vi "Actor Core.vi"(8 "error in":errorcluster, 11 "gController in":refnum<class "gController.lvclass">) -> (0 "error out":errorcluster, 3 "Actor out":refnum<class "Actor.lvclass">)   [LabVIEW 2017, in "Controller.lvlib" / "gController.lvclass"]
doc: "(<B>Filename</B>: Actor Framework.lvlib:Actor.lvclass:Actor Core.vi)\n\nReceives messages to the actor, reacts to them, and initiates any error handling that may shut the actor down.\n\nDescendant classes may override this VI to append parallel tasks for the actor to complete while it handles messages. Overrides use the Call Parent Method node."
uses:
  gController.lvclass
  C:/Program Files (x86)/National Instruments/LabVIEW 2017/vi.lib/MSR Consulting, LLC/General Reuse/SuperActor/SuperActor.lvclass
  <vilib>/ActorFramework/Actor/Actor.lvclass
  File Actor/File Actor.lvclass
  C:/Program Files (x86)/National Instruments/LabVIEW 2017/vi.lib/ActorFramework/Actor/Actor.lvclass
  File Actor/Messages/Abstract/Saving File Message/Saving File Message.lvclass
  Commands/Exe Write Main CMD/Exe Write Main CMD.lvclass
  G:/sw_repo/For Builds/Nicholas/File Actor/Messages/Abstract/Exe Write/Exe Write.lvclass
  <vilib>/ActorFramework/Message Enqueuer/Message Enqueuer.lvclass
  <vilib>/Platform/TimedLoop/XDataNode/timing_clust.ctl
  <vilib>/Platform/TimedLoop/XDataNode/nitl_modes.ctl
  <vilib>/Platform/TimedLoop/XDataNode/wakeup.ctl
  <vilib>/MSR Consulting, LLC/General Reuse/SuperActor/SuperActor.lvclass/SuperActor.ctl
  gController.lvclass/gController.ctl
  Commands/Exe Write Main CMD/Exe Write Main CMD.lvclass/Exe Write Main CMD.ctl
  File Actor/File Actor.lvclass/File Actor.ctl
  File Actor/Messages/To/Data/File Data Message.lvclass
  C:/Program Files (x86)/National Instruments/LabVIEW 2017/vi.lib/ActorFramework/Message/Message.lvclass
  <vilib>/ActorFramework/Message Enqueuer/Message Enqueuer.lvclass/Message Enqueuer.ctl
  File Actor/Write Saving FIle MSG.vi
  File Actor/Write Exe Write.vi
  <vilib>/MSR Consulting, LLC/General Reuse/SuperActor/Write ID.vi
  File Actor/Write Cfg Header.vi
  File Actor/Write Wait on Registration_.vi
  <vilib>/MSR Consulting, LLC/General Reuse/SuperActor/Read Log Session.vi
  Read DataMap.vi
  Commands/Exe Write Main CMD/Write DataMap.vi
  <vilib>/MSR Consulting, LLC/General Reuse/SuperActor/Read EnqueuerMap.vi
  <vilib>/ActorFramework/Message Priority Queue/Priority Enqueue.vi
  File Actor/Write Registration Complete.vi
  <vilib>/Platform/TimedLoop/XDataNode/XDataNode.xnode
  <vilib>/MSR Consulting, LLC/General Reuse/Session APIs/_Session Fwk/Session - Root.lvclass
  <vilib>/MSR Consulting, LLC/General Reuse/SuperActor/SuperActor.lvclass
  <vilib>/MSR Consulting, LLC/General Reuse/Session APIs/Session Log/System Log.lvclass
  <vilib>/Platform/TimedLoop/XDataNode/XDNodeRunTimeDep.lvlib
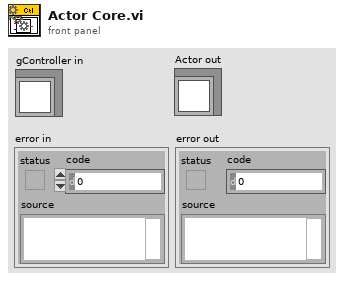
[diagram p1: front panel]
types:
  T1 = typedef "Session - Root.lvclass/Session Handle.ctl" = refnum<data-value>
  T2 = typedef "XDNodeRunTimeDep.lvlib/timing_clust.ctl" = cluster{"Expected End [f-1]":u64, "Actual End [f-1]":u64, "Finished Late? [f-1]":bool, "Expected End [i-1]":u64, "Actual End [i-1]":u64, "Finished Late? [i-1]":bool, "Expected Start [i]":u64, "Actual Start [i]":u64, "Expected Start [f]":u64, "Actual Start [f]":u64, "Source Name":string, "Structure Name":string, "Period":i64, "Deadline":i64, "Offset":i64, "Start":i64, "Priority":i32, "Timeout":i32, "Mode":T3, "Wakeup Reason":T4, "Error":errorcluster, "Source Type":string, "Secondary Source Type":string, "Global End Time":u64, "Global Start Time":u64, "Frame Duration":u64, "Iteration Duration":u64, "Assigned CPU":i32, "I/O Scan Engine Mode":u32}
  T3 = typedef "XDNodeRunTimeDep.lvlib/nitl_modes.ctl" = enum32{"No Change", "Process missed periods, maintain original phase", "Discard missed periods, maintain original phase", "Process missed periods, ignore original phase", "Discard missed periods, ignore original phase"}
  T4 = typedef "XDNodeRunTimeDep.lvlib/wakeup.ctl" = enum32{"Normal", "Aborted", "Asynchronous wakeup", "Timing source error", "Timed loop error", "Timeout"}
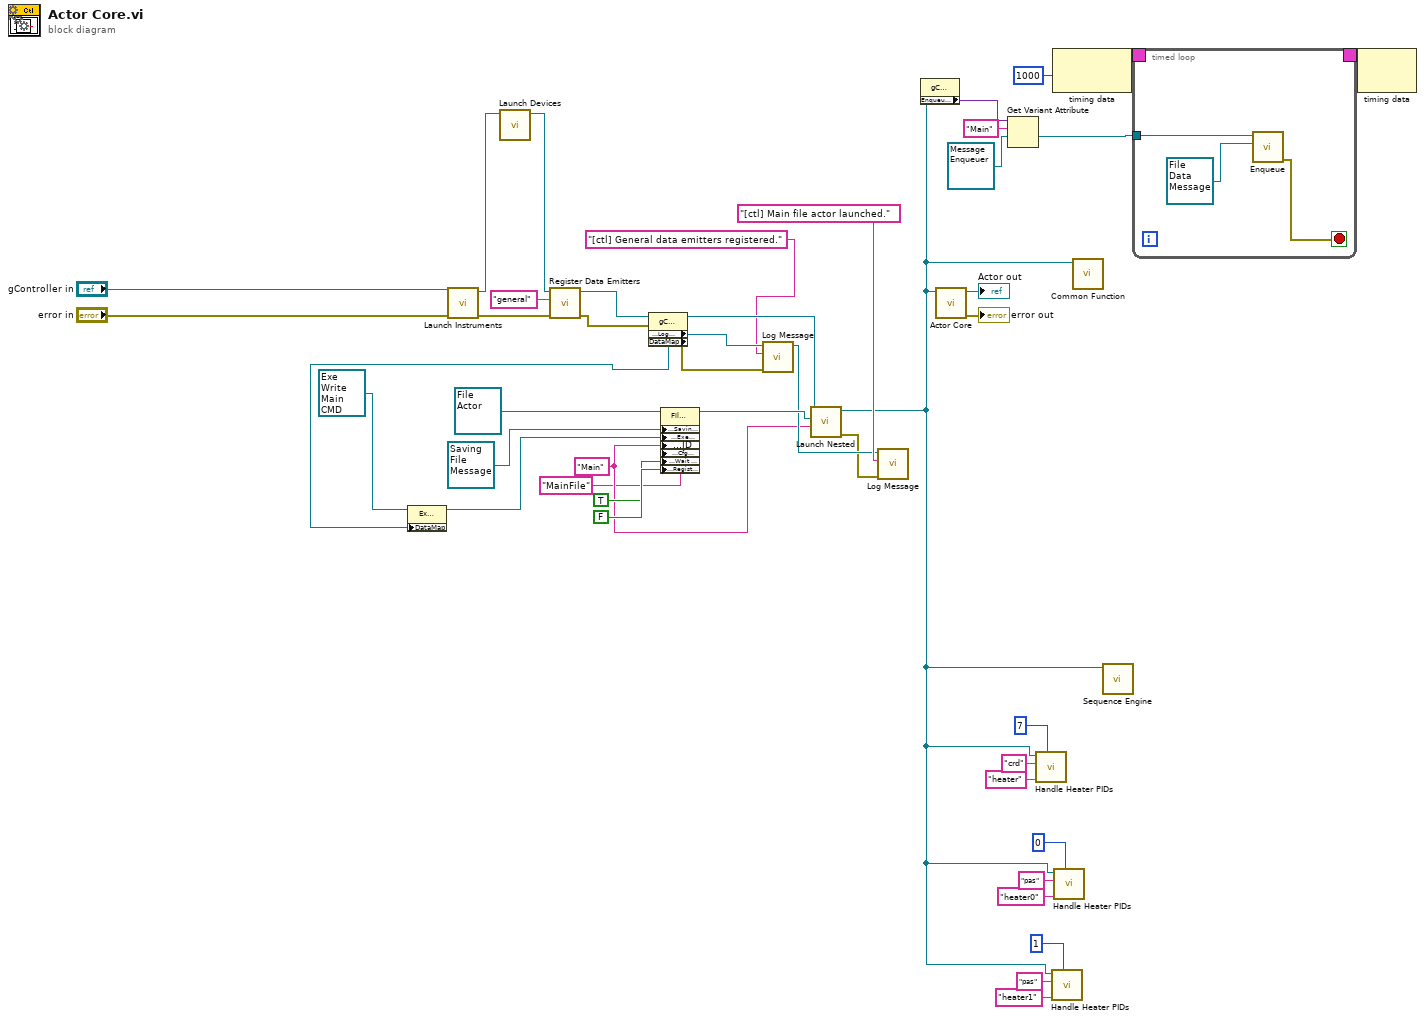
[diagram p0: block diagram]
diagram:
  w24 = "Main" ("ID")
  n1 = call "Launch Instruments.vi"("error in (no error)"="error in", "gController in"="gController in") -> ("error out"=w42:errorcluster, "gController out"=w43:refnum<class "gController.lvclass">)  [unwired: 8 in]
  n2 = call "Launch Devices.vi"("gController in"=w43) -> ("gController out"=w40:refnum<class "gController.lvclass">)  [unwired: 10 in]
  n3 = call "Register Data Emitters.vi"("error in"=w42, "Emitter"="general", "gController in"=w40) -> ("error out"=w29:errorcluster, "gController out"=w33:refnum<class "gController.lvclass">)  [unwired: 7 in]
  n4 = property class="gController"(reference=w33, error in=w29) -> (reference out=w32:refnum<class "gController.lvclass">, error out=w28:errorcluster, "Accessors:Log Session"=w31:T1, "DataMap"=w20:refnum<data-value>)
  n5 = property class="Exe Write Main CMD.lvclass"(reference=refnum<class "Exe Write Main CMD.lvclass"> refnum ("Controller.lvlib:Exe Write Main CMD.lvclass"), "DataMap"=w20) -> (reference out=w21:refnum<class "Exe Write Main CMD.lvclass">)  [unwired: 1 in, 1 out]
  n6 = property class="File Actor"(reference=refnum<class "File Actor.lvclass"> refnum ("File Library.lvlib:File Actor"), "Accessors:Saving FIle MSG"=refnum<class "Saving File Message.lvclass"> refnum ("File Library.lvlib:Saving Main File MSG"), "Accessors:Exe Write"=w21, "Accessors:ID"=w24, "Accessors:Cfg Header"="MainFile" ("Cfg Header"), "Accessors:Wait on Registration_"=TRUE ("Wait on Registration_"), "Accessors:Registration Complete"=FALSE ("Registration Complete")) -> (reference out=w34:refnum<class "File Actor.lvclass">)  [unwired: 1 in, 1 out]
  n7 = call <vilib>:"Log Message.vi"("error in"=w28, "MSG In"="[ctl] General data emitters registered." ("format string"), "session in"=w31) -> ("session out"=w26:T1)  [unwired: 7 in, 1 out]
  n8 = call <vilib>:"Launch Nested.vi"("ID"=w24, "Nested Actor"=w34, "SuperActor in"=w32) -> ("error out"=w25:errorcluster, "SuperActor out"=w10:refnum<class "gController.lvclass">)  [unwired: 6 in, 1 out]
  n9 = call <vilib>:"Log Message.vi"("error in"=w25, "MSG In"="[ctl] Main file actor launched." ("format string"), "session in"=w26) -> ()  [unwired: 7 in, 2 out]
  n10 = property class="gController"(reference=w10) -> ("EnqueuerMap"=w19:variant)  [unwired: 1 in, 2 out]
  n11 = call-parent "Actor Core.vi"("Actor in"=w10) -> ("error out"=→"error out":errorcluster, "Actor out"=→"Actor out":refnum<class "Actor.lvclass">)  [unwired: 9 in]
  n12 = Get Variant Attribute(Variant=w19, name="Main", default value (empty Variant)=refnum<class "Message Enqueuer.lvclass"> refnum ("Nested Actor's Enqueuer")) -> (value=w14:refnum<class "Message Enqueuer.lvclass">)  [unwired: 1 in, 3 out]
  n13 = call "Handle Heater PIDs.vi"("DataIndex"=7, "Subtag"="heater", "HeaterTag"="crd", "gController in"=w10) -> ()  [unwired: 8 in]
  n14 = call "Handle Heater PIDs.vi"("DataIndex"=1, "Subtag"="heater1", "HeaterTag"="pas", "gController in"=w10) -> ()  [unwired: 8 in]
  n15 = node-c288(i64 1000 ("Period")) -> (w16:T2)
  n16 = call "Handle Heater PIDs.vi"("DataIndex"=0, "Subtag"="heater0", "HeaterTag"="pas", "gController in"=w10) -> ()  [unwired: 8 in]
  n17 = call "Common Function.vi"("gController in"=w10) -> ()  [unwired: 11 in]
  n18 = call "Sequence Engine.vi"("gController in"=w10) -> ()  [unwired: 10 in, 1 out]
  n19 = timed-loop {
    timing: w16 -> [_]
    timing-out: [_] -> w15
    tunnel: w14 -> [w47]
    stop <- w45 stop-if-true
    n20 = call <vilib>:"Enqueue.vi"("Message"=refnum<class "File Data Message.lvclass"> refnum ("File Library.lvlib:File Data MSG"), "Message Enqueuer in"=w47) -> ("error out"=w45:errorcluster)  [unwired: 8 in, 1 out]
  }
  n21 = node-c288(w15) -> ()  [unwired: 1 out]
